vi "FocalSpot.vi"(7 "Racine chemin de sauvegarde":path=path "C:/Users/loa/Documents/DONNEES MANIP GAZ/Hiver 2015") -> ()   [LabVIEW 2014]
uses:
  <vilib>/addons/PixeLINK/Low Level Functions/ACQUISITION.llb/TDPU-Acquisition-StreamState.ctl
  <vilib>/addons/PixeLINK/Low Level Functions/CAMERA_FEATURES.llb/TDPU-CameraFeatures-FeatureIds.ctl
  <vilib>/addons/PixeLINK/Low Level Functions/CAMERA_FEATURES.llb/TDPU-CameraFeatures-FeatureFlags.ctl
  <vilib>/Platform/TimedLoop/XDataNode/timing_clust.ctl
  <vilib>/Platform/TimedLoop/XDataNode/nitl_modes.ctl
  <vilib>/Platform/TimedLoop/XDataNode/wakeup.ctl
  <vilib>/platform/TimedLoop/XDataNode/XDataNode.xnode
  <vilib>/Platform/TimedLoop/XDataNode/XDNodeRunTimeDep.lvlib
panel:
  in  "Transmission":dbl=0.5
  out "Intensity (measured)\nx10^18 W/cm²":dbl=2.0
  out "Div":dbl
  in  "Automatic\nfolder naming":bool=TRUE
  in  "Imager":u32(ring) items=["Cam 0"=953000197]
  out "?":dbl[][](graph)
  out "?":dbl[][](graph)
  in  "Background \nsubstraction":bool
  out "Intensity (gaussian)\nx10^18 W/cm²":dbl=2.0
  out "Peak power (TW)":dbl=2.0
  out "FWHM y (µm)":dbl=2.0
  out "FWHM x (µm)":dbl=2.0
  in  "Duration FWHM (fs)":dbl=4.5
  in  "Pulse Energy (mJ)":dbl=5.0
  in  "Calibration µm/px":dbl=0.5
  out "Error OUT 2":errorcluster
  out "Error OUT":errorcluster
  out "Saturating?":bool
  out "Average":dbl
  out "Std Dev":dbl
  in  "Overwrite?":bool
  in  "Snap current Data":bool
  in  "Save Data":bool
  out "Warning":bool
  out "Message":string
  in  "Indice":u32
  in  "Nom du fichier":string="tir"
  in  "Mode de Sauvegarde":u16(ring)=1 items=["Manuel", "Automatique"]
  out "Max Val":u16
  out "Captured Image":dbl[][](graph)
  out "Waiting for Trigger":bool
  in  "Continuous Grab":bool
  in  "Snap Next frame":bool
  out "Camera Handle":u32
  in  "Stop Grab\n(Insistez!)":bool
  in  "Trigger Type":enum16{"Free Running", "Software", "Hardware"}(ring)
  in  "Trigger Polarity":enum16{"Positive", "Negative"}(ring)
  in  "Refresh Trigger":bool
  in  "Exposure Time":dbl(slide) min=6.350000330712646e-05 max=10.0 scale=6.350000330712646e-05..10.0
  in  "stop":bool
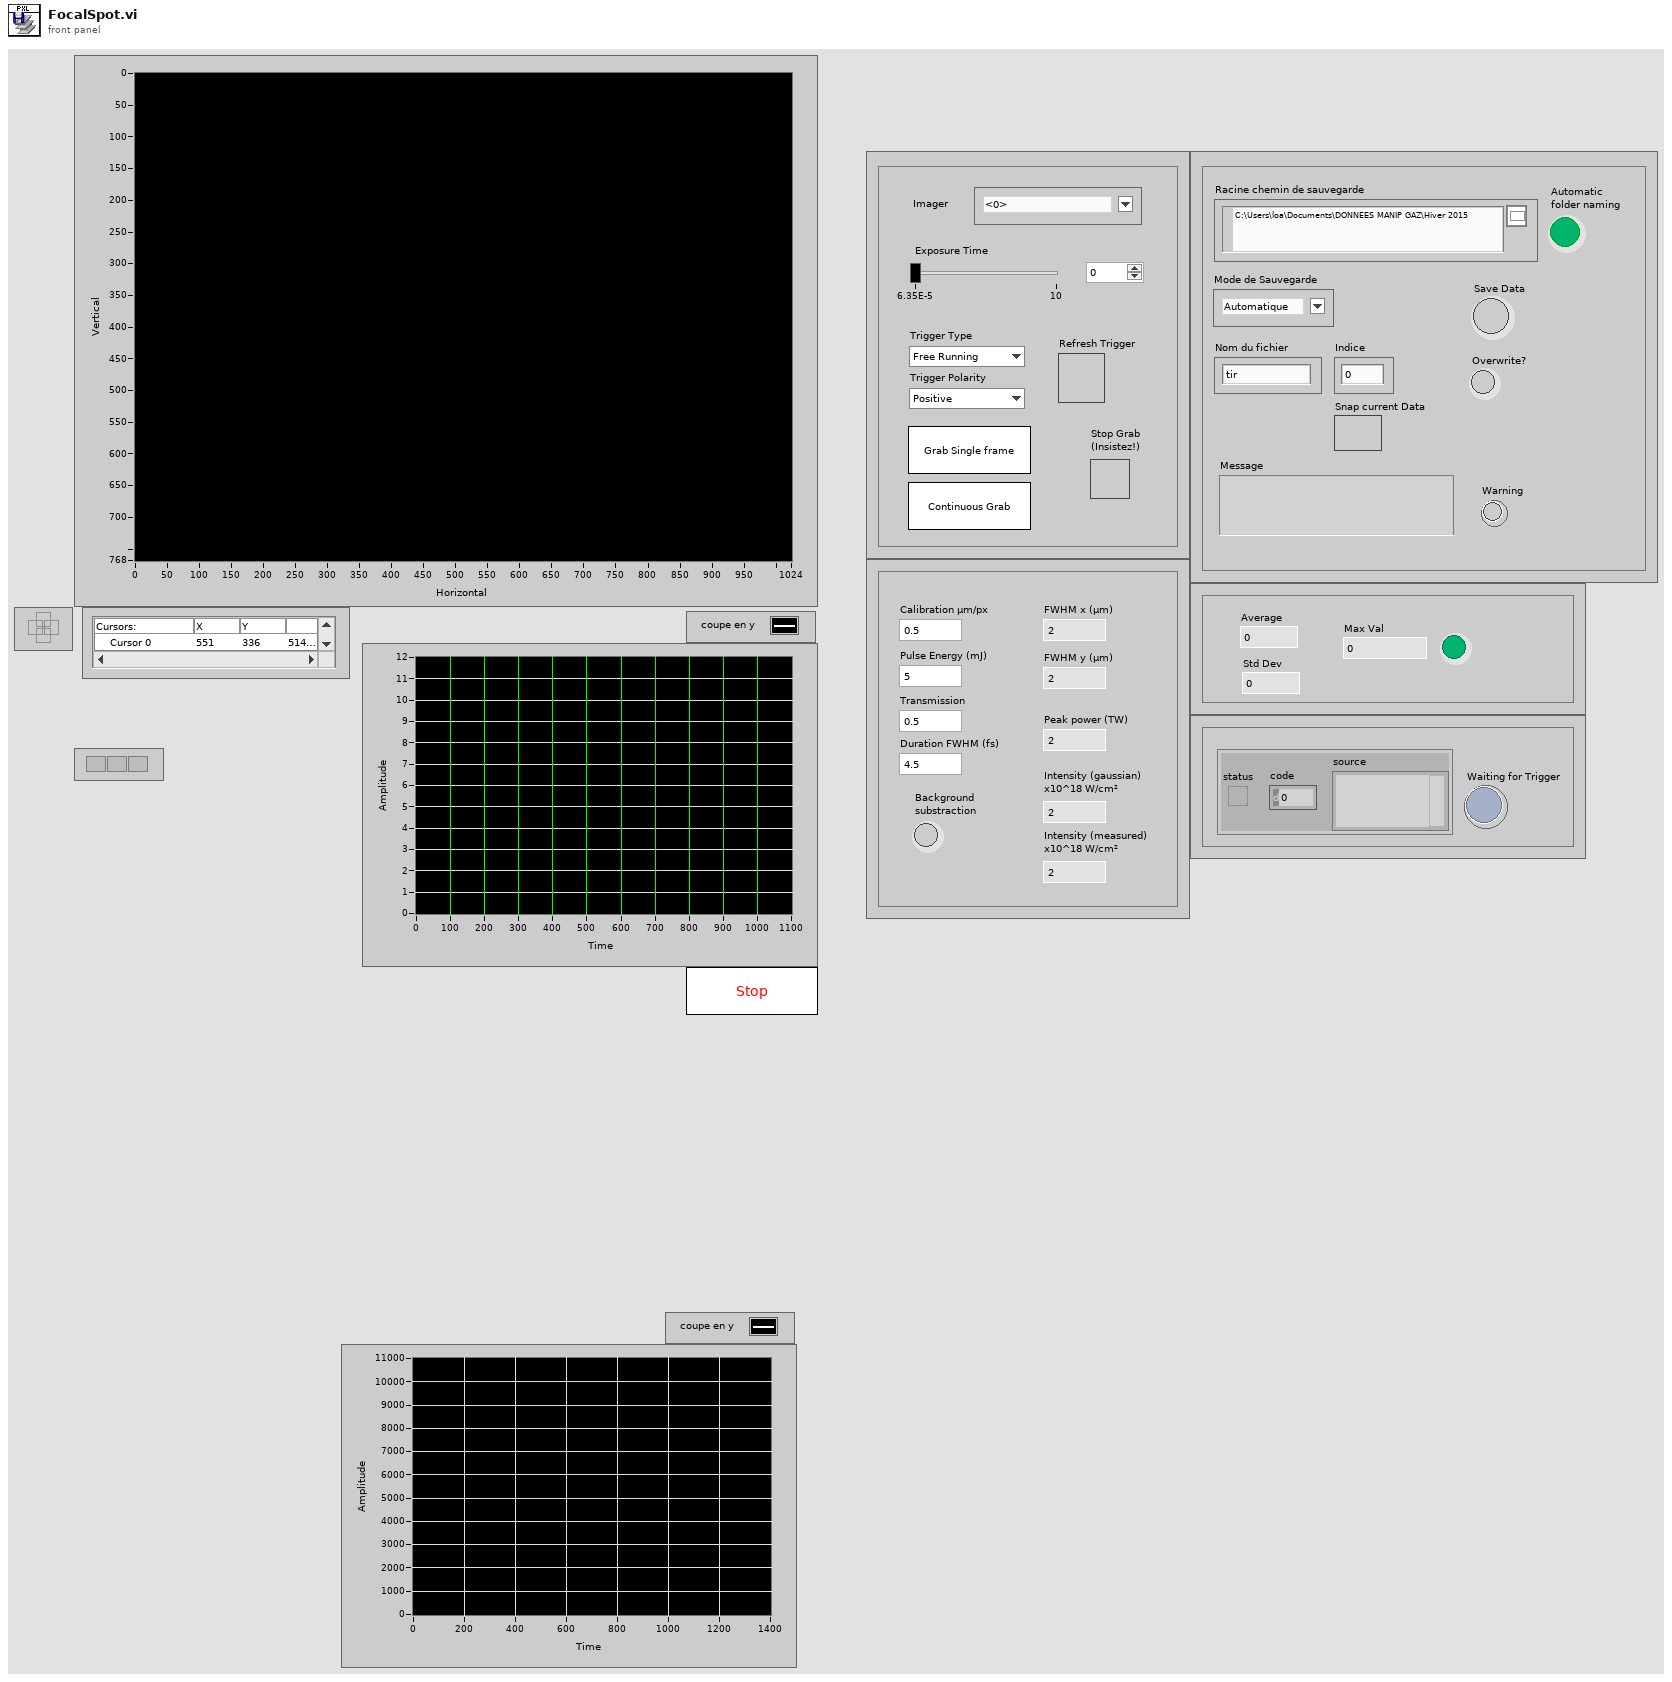
[diagram p1: front panel]
types:
  T1 = typedef "TDPU-Acquisition-StreamState.ctl" = u32
  T2 = typedef "TDPU-CameraFeatures-FeatureFlags.ctl" = u32
  T3 = typedef "TDPU-CameraFeatures-FeatureIds.ctl" = u32
  T4 = typedef "XDNodeRunTimeDep.lvlib/timing_clust.ctl" = cluster{"Expected End [f-1]":u64, "Actual End [f-1]":u64, "Finished Late? [f-1]":bool, "Expected End [i-1]":u64, "Actual End [i-1]":u64, "Finished Late? [i-1]":bool, "Expected Start [i]":u64, "Actual Start [i]":u64, "Expected Start [f]":u64, "Actual Start [f]":u64, "Source Name":string, "Structure Name":string, "Period":i64, "Deadline":i64, "Offset":i64, "Start":i64, "Priority":i32, "Timeout":i32, "Mode":T5, "Wakeup Reason":T6, "Error":errorcluster, "Source Type":string, "Secondary Source Type":string, "Global End Time":u64, "Global Start Time":u64, "Frame Duration":u64, "Iteration Duration":u64, "Assigned CPU":i32, "I/O Scan Engine Mode":u32}
  T5 = typedef "XDNodeRunTimeDep.lvlib/nitl_modes.ctl" = enum32{"No Change", "Process missed periods, maintain original phase", "Discard missed periods, maintain original phase", "Process missed periods, ignore original phase", "Discard missed periods, ignore original phase"}
  T6 = typedef "XDNodeRunTimeDep.lvlib/wakeup.ctl" = enum32{"Normal", "Aborted", "Asynchronous wakeup", "Timing source error", "Timed loop error", "Timeout"}
  T7 = typedef "LVStringsAndValuesArrayTypeDef_U32.ctl" = cluster{"String":string, "Value":u32}[]
  T8 = typedef "TDPU-Identification-Camera_Info.ctl" = cluster{"VendorName":string, "ModelName":string, "Description":string, "SerialNumber":string, "FirmwareVersion":string, "FPGAVersion":string, "CameraName":string}
  T9 = typedef "TDPU-Acquisition-Frame_Desc.ctl" = cluster{"uSize":u32, "fFrameTime":dbl, "uFrameNumber":u32, "Brightness":cluster{"fValue":dbl}, "AutoExposure":cluster{"fValue":dbl}, "Sharpness":cluster{"fValue":dbl}, "WhiteBalance":cluster{"fValue":dbl}, "Hue":cluster{"fValue":dbl}, "Saturation":cluster{"fValue":dbl}, "Gamma":cluster{"fValue":dbl}, "Shutter":cluster{"fValue":dbl}, "Gain":cluster{"fValue":dbl}, "Iris":cluster{"fValue":dbl}, "Focus":cluster{"fValue":dbl}, "Temperature":cluster{"fValue":dbl}, "Trigger":cluster{"fMode":dbl, "fType":dbl, "fPolarity":dbl, "fDelay":dbl, "fParameter":dbl}, "Zoom":cluster{"fValue":dbl}, "Pan":cluster{"fValue":dbl}, "Tilt":cluster{"fValue":dbl}, "OpticalFilter":cluster{"fValue":dbl}, "GPIO":cluster{"fMode":dbl[], "fPolarity":dbl[], "fParameter1":dbl[], "fParameter2":dbl[], "fParameter3":dbl[]}, "FrameRate":cluster{"fValue":dbl}, "ROI":cluster{"fLeft":dbl, "fTop":dbl, "fWidth":dbl, "fHeight":dbl}, "Flip":cluster{"fHorizontal":dbl, "fVertical":dbl}, "PixelAddressingValue":cluster{"fValue":dbl}, "PixelFormat":cluster{"fValue":dbl}, "ExtendedShutter":cluster{"fKneePoint":dbl[]}, "AutoROI":cluster{"fLeft":dbl, "fTop":dbl, "fWidth":dbl, "fHeight":dbl}, "WhiteShading":cluster{"fRedGain":dbl, "fGreenGain":dbl, "fBlueGain":dbl}, "Rotate":cluster{"fValue":dbl}, "PixelAddressingMode":cluster{"fValue":dbl}}
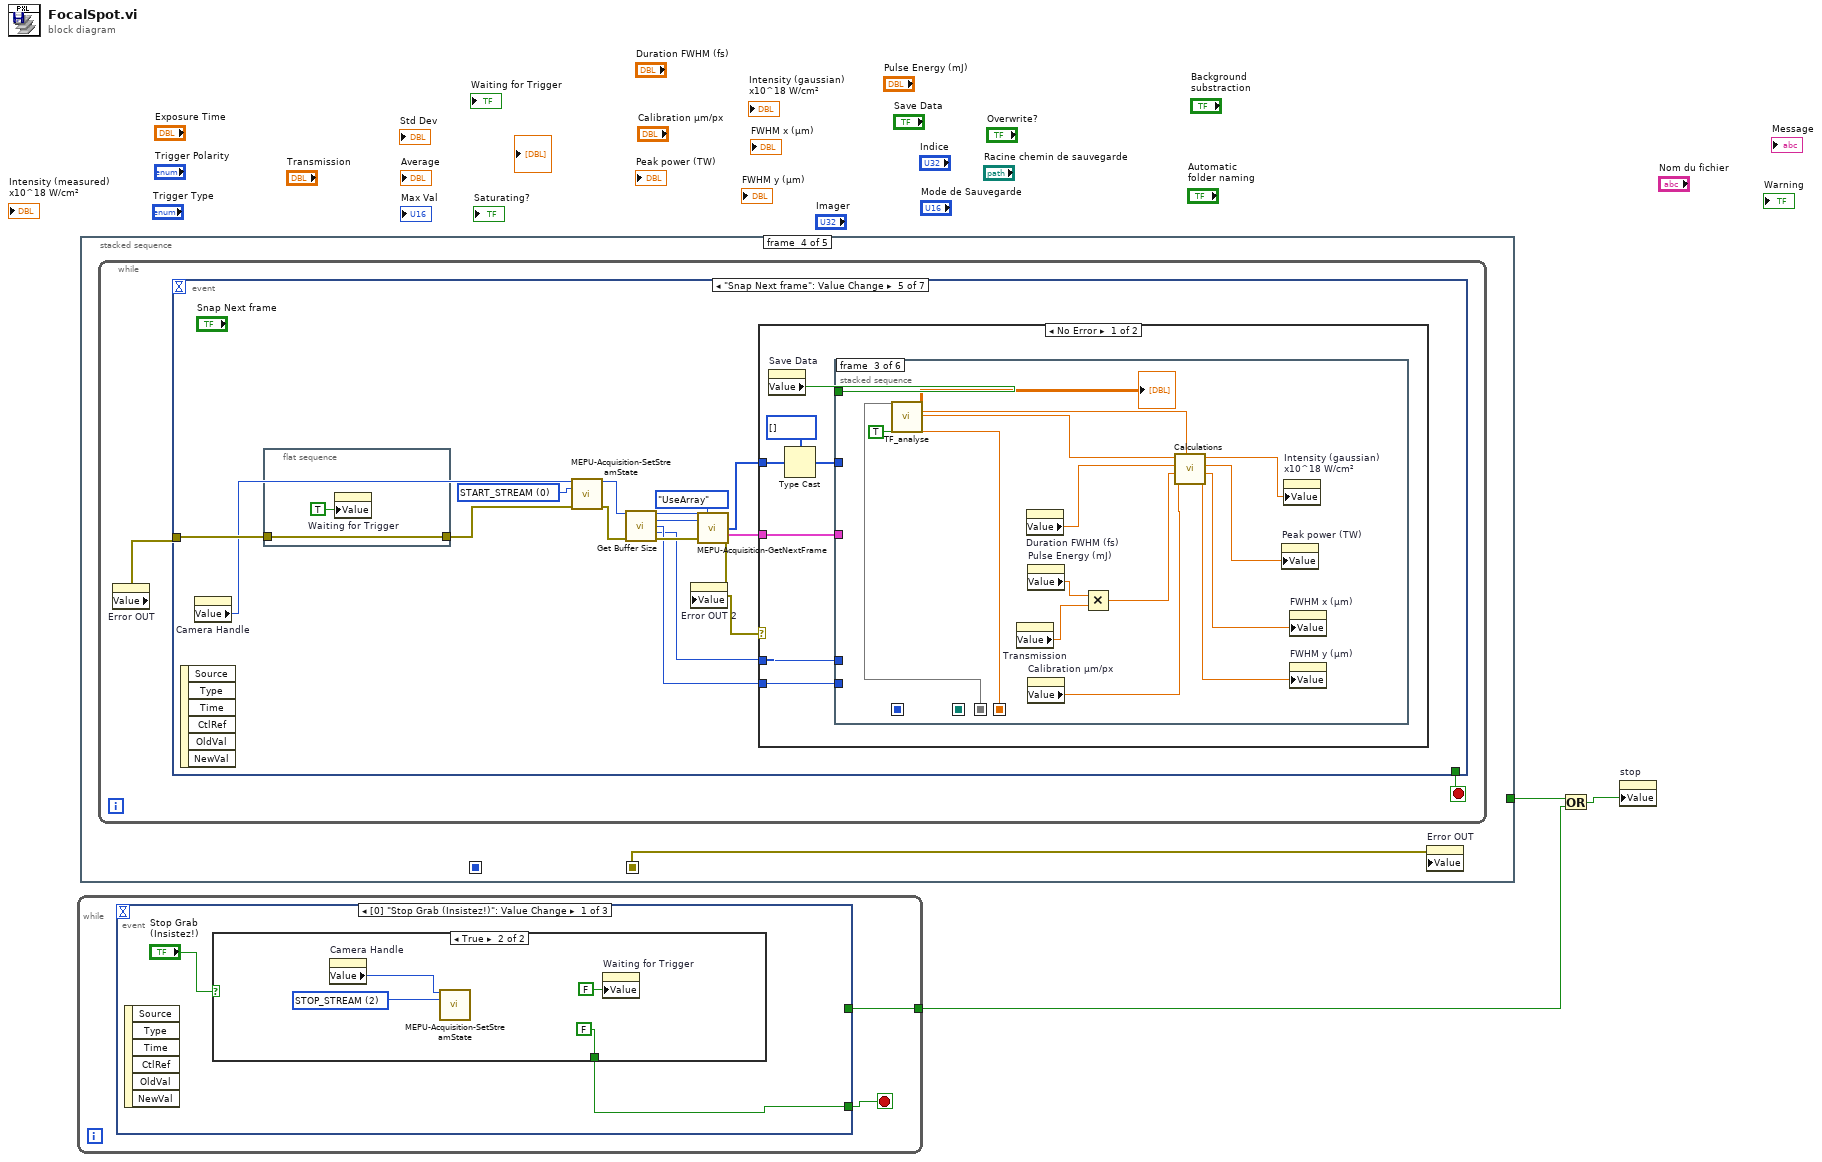
[diagram p0: block diagram]
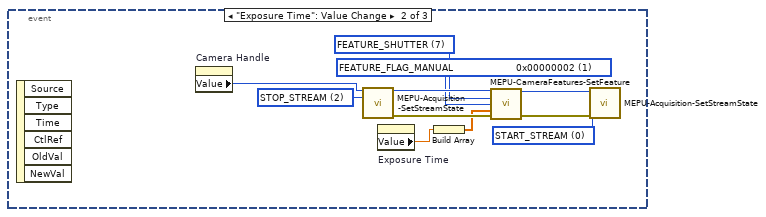
[diagram p3: hidden frame]
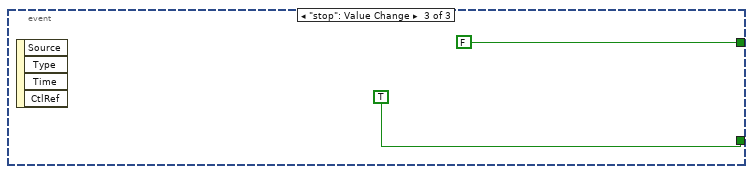
[diagram p4: hidden frame]
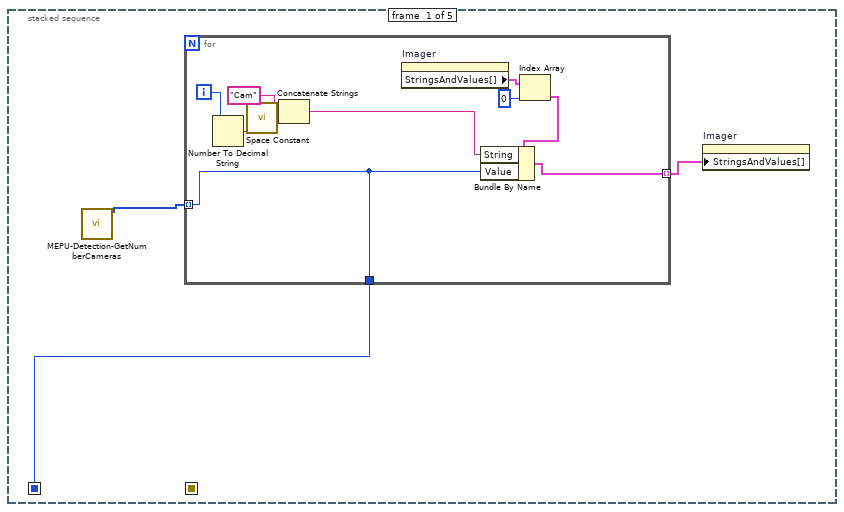
[diagram p5: hidden frame]
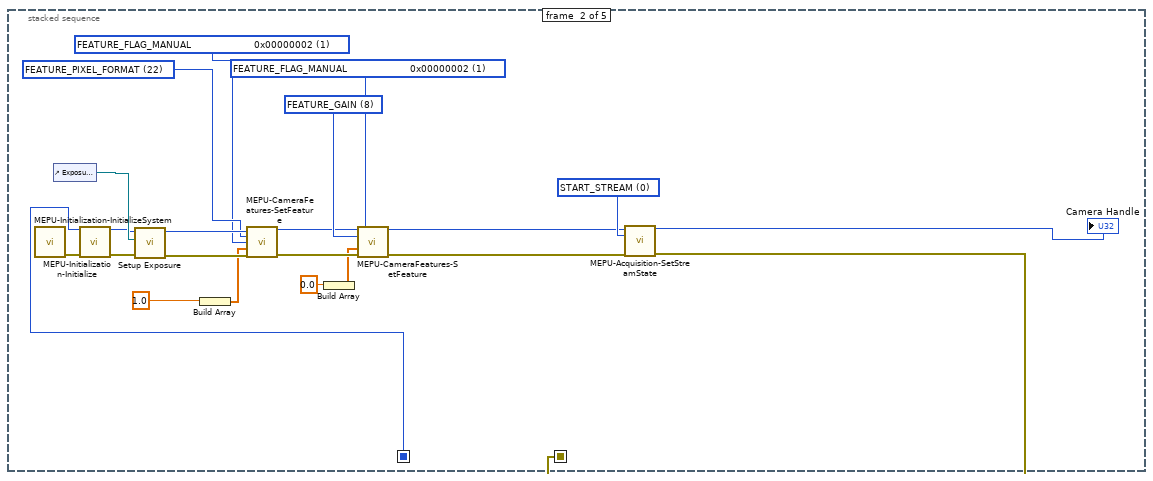
[diagram p6: hidden frame]
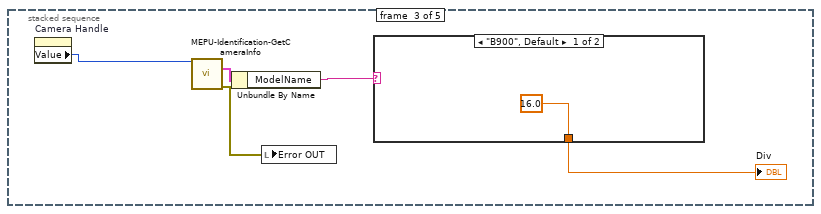
[diagram p7: hidden frame]
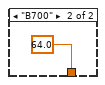
[diagram p8: hidden frame]
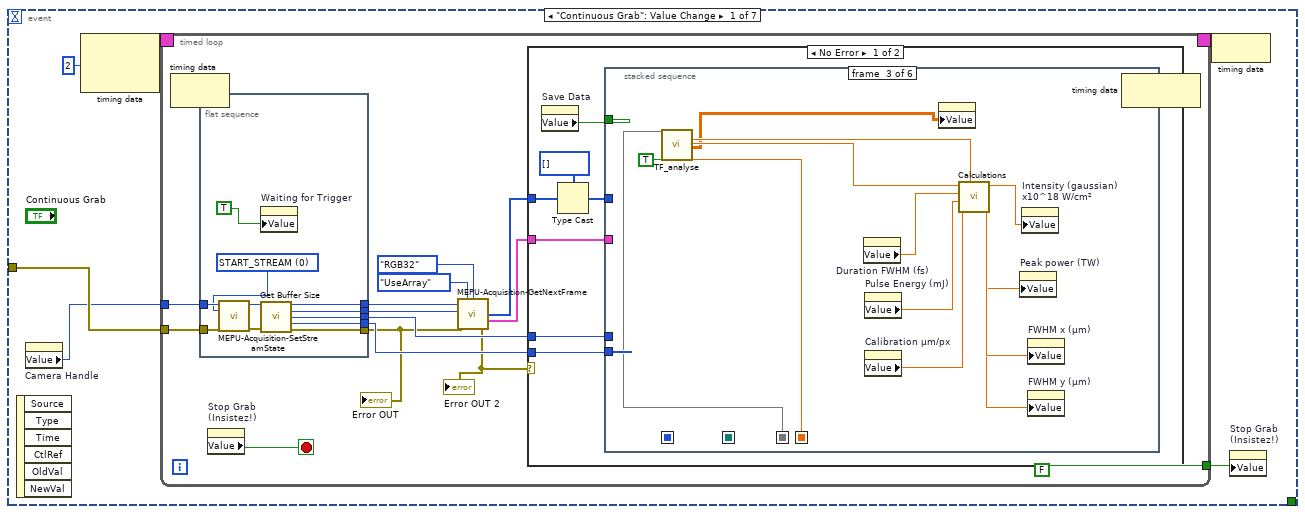
[diagram p9: hidden frame]
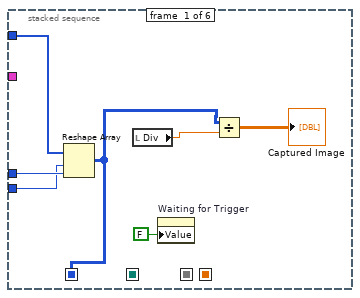
[diagram p10: hidden frame]
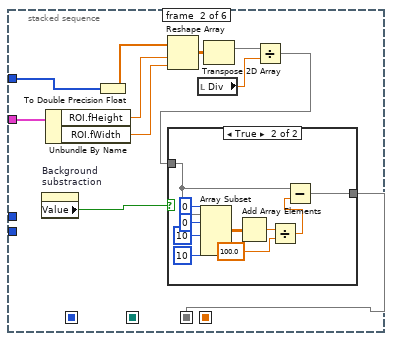
[diagram p11: hidden frame]
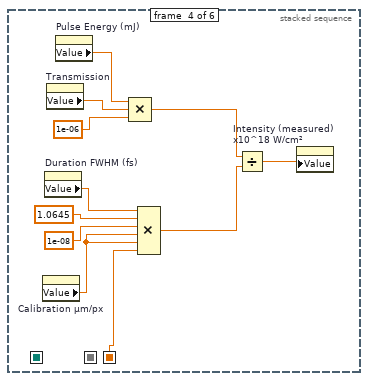
[diagram p13: hidden frame]
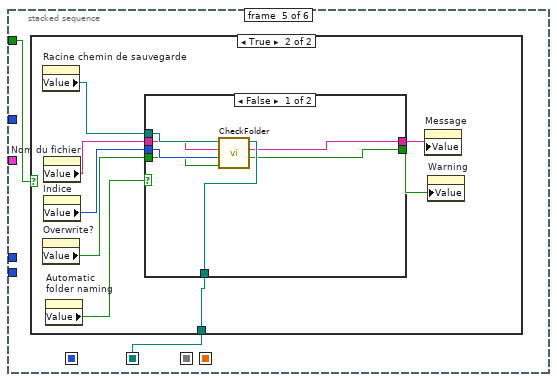
[diagram p14: hidden frame]
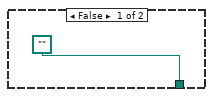
[diagram p15: hidden frame]
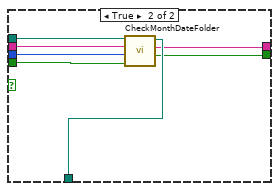
[diagram p16: hidden frame]
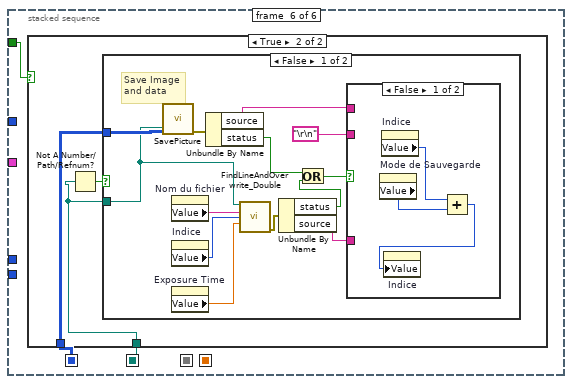
[diagram p17: hidden frame]
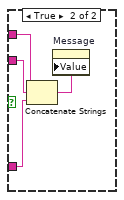
[diagram p19: hidden frame]
diagram:
  n1 = while {
    tunnel: [w4] -> w2
    stop <- w5 stop-if-true
    n2 = event shown="[0] \"Stop Grab (Insistez!)\": Value Change" {
      selector: _ -> [_ _ _]
      dyn-events: _ -> [_ _ _]
      timeout: _ -> [_ _ _]
      tunnel: [w6 _ TRUE] -> w5
      tunnel: [_ _ FALSE] -> w4
      event "Stop Grab\n(Insistez!)": Value Change {
        n3 = event-data() -> ()  [unwired: 1 in, 6 out]
        n4 = case shown="True" "Stop Grab\n(Insistez!)" {
          tunnel: [_ FALSE] -> w6
          frame False {
          }
          frame True {
            w11 = T1 2 items=["START_STREAM", "PAUSE_STREAM", "STOP_STREAM"] ("uStreamState IN")
            n5 = property on="Camera Handle" class="DigNum (strict)"() -> ("Value"=w9:u32)  [unwired: 2 in, 2 out]
            n6 = call <vilib>:"MEPU-Acquisition-SetStreamState.vi"("hCamera IN"=w9, "uStreamState IN"=w11) -> ()  [unwired: 12 in, 2 out]
            n7 = property on="Waiting for Trigger" class="Bool (strict)"("Value"=FALSE ("Waiting for Trigger")) -> ()  [unwired: 2 in, 2 out]
          }
        }
      }
      event "Exposure Time": Value Change {
        w22 = T1 0 items=["START_STREAM", "PAUSE_STREAM", "STOP_STREAM"] ("uStreamState IN")
        w21 = T1 2 items=["START_STREAM", "PAUSE_STREAM", "STOP_STREAM"] ("uStreamState IN")
        w14 = T2 1 items=["FEATURE_FLAG_PRESENCE                 0x00000001", "FEATURE_FLAG_MANUAL                     0x00000002", "FEATURE_FLAG_AUTO                         0x00000004", "FEATURE_FLAG_ONEPUSH                   0x00000008", "FEATURE_FLAG_OFF                            0x00000010", "FEATURE_FLAG_DESC_SUPPORTED    0x00000020", "FEATURE_FLAG_READ_ONLY               0x00000040"] ("uFlags IN")
        w13 = T3 7 items=["FEATURE_BRIGHTNESS", "FEATURE_EXPOSURE", "FEATURE_SHARPNESS", "FEATURE_WHITE_BAL", "FEATURE_HUE", "FEATURE_SATURATION", "FEATURE_GAMMA", "FEATURE_SHUTTER", "FEATURE_GAIN", "FEATURE_IRIS", "FEATURE_FOCUS", "FEATURE_TEMPERATURE", "FEATURE_TRIGGER", "FEATURE_ZOOM", "FEATURE_PAN", "FEATURE_TILT", "FEATURE_OPT_FILTER", "FEATURE_GPIO", "FEATURE_FRAME_RATE", "FEATURE_ROI", "FEATURE_FLIP", "FEATURE_PIXEL_ADDRESSING", "FEATURE_PIXEL_FORMAT", "FEATURE_EXTENDED_SHUTTER", "FEATURE_AUTO_ROI", "FEATURE_LOOKUP_TABLE", "FEATURE_MEMORY_CHANNEL", "FEATURE_WHITE_SHADING", "FEATURE_ROTATE", "FEATURE_IMAGER_CLK_DIVISOR", "FEATURE_TRIG_WITH_CNTRLD_LIGHT", "FEATURE_MAX_PIXEL_SIZE"] ("uFeatureId IN")
        n8 = event-data() -> ()  [unwired: 1 in, 6 out]
        n9 = property on="Camera Handle" class="DigNum (strict)"() -> ("Value"=w12:u32)  [unwired: 2 in, 2 out]
        n10 = call <vilib>:"MEPU-Acquisition-SetStreamState.vi"("hCamera IN"=w12, "uStreamState IN"=w21) -> ("hCamera OUT"=w17:u32, "Error OUT"=w20:errorcluster)  [unwired: 12 in]
        n11 = property on="Exposure Time" class="Slide (strict)"() -> ("Value"=w15:dbl)  [unwired: 2 in, 2 out]
        n12 = Build Array(w15) -> (w16:dbl[])
        n13 = call <vilib>:"MEPU-CameraFeatures-SetFeature.vi"("hCamera IN"=w17, "uFeatureId IN"=w13, "uFlags IN"=w14, "pParms IN"=w16, "Error IN"=w20) -> ("hCamera OUT"=w18:u32, "Error OUT"=w19:errorcluster)  [unwired: 9 out]
        n14 = call <vilib>:"MEPU-Acquisition-SetStreamState.vi"("hCamera IN"=w18, "uStreamState IN"=w22, "Error IN"=w19) -> ()  [unwired: 11 in, 2 out]
      }
      event "stop": Value Change {
        n15 = event-data() -> ()  [unwired: 1 in, 4 out]
      }
    }
  }
  n16 = stacked-sequence {
    seq-local: [_ w48 _ _ _] -> [_ _ _ w67 _]
    seq-local: [w25 _ _ _ _] -> [_ w38 _ _ _]
    tunnel: [_ _ _ _ TRUE] -> w3
    frame #0 {
      n17 = call <vilib>:"MEPU-Detection-GetNumberCameras.vi"() -> ("LV_SerialNumbers OUT"=w27:u32[])  [unwired: 13 in, 2 out]
      n18 = for {
        tunnel: w27 -> [w28] mode=indexing
        tunnel: [w33] -> w26 mode=indexing
        tunnel: [w28] -> w25
        i -> [w31]
        n19 = Number To Decimal String(number=w31) -> (decimal integer string=w29:string)  [unwired: 1 in]
        n20 = call <vilib>:"Space Constant.vi"() -> ("String"=w30:string)
        n21 = Concatenate Strings("Cam", w30, w29) -> (w34:string)
        n22 = property on="Imager" class="Ring (strict)"() -> ("StringsAndValues[]"=w37:T7)  [unwired: 2 in, 2 out]
        n23 = Index Array(array=w37, index=0) -> (element=w35:cluster{"String":string, "Value":u32})
        n24 = Bundle By Name(cluster=w35, "String"=w34, "Value"=w28) -> (w33:cluster{"String":string, "Value":u32})
      }
      n25 = property on="Imager" class="Ring (strict)"("StringsAndValues[]"=w26) -> ()  [unwired: 2 in, 2 out]
    }
    frame #1 {
      w43 = T2 1 items=["FEATURE_FLAG_PRESENCE                 0x00000001", "FEATURE_FLAG_MANUAL                     0x00000002", "FEATURE_FLAG_AUTO                         0x00000004", "FEATURE_FLAG_ONEPUSH                   0x00000008", "FEATURE_FLAG_OFF                            0x00000010", "FEATURE_FLAG_DESC_SUPPORTED    0x00000020", "FEATURE_FLAG_READ_ONLY               0x00000040"] ("uFlags IN")
      w42 = T3 8 items=["FEATURE_BRIGHTNESS", "FEATURE_EXPOSURE", "FEATURE_SHARPNESS", "FEATURE_WHITE_BAL", "FEATURE_HUE", "FEATURE_SATURATION", "FEATURE_GAMMA", "FEATURE_SHUTTER", "FEATURE_GAIN", "FEATURE_IRIS", "FEATURE_FOCUS", "FEATURE_TEMPERATURE", "FEATURE_TRIGGER", "FEATURE_ZOOM", "FEATURE_PAN", "FEATURE_TILT", "FEATURE_OPT_FILTER", "FEATURE_GPIO", "FEATURE_FRAME_RATE", "FEATURE_ROI", "FEATURE_FLIP", "FEATURE_PIXEL_ADDRESSING", "FEATURE_PIXEL_FORMAT", "FEATURE_EXTENDED_SHUTTER", "FEATURE_AUTO_ROI", "FEATURE_LOOKUP_TABLE", "FEATURE_MEMORY_CHANNEL", "FEATURE_WHITE_SHADING", "FEATURE_ROTATE", "FEATURE_IMAGER_CLK_DIVISOR", "FEATURE_TRIG_WITH_CNTRLD_LIGHT", "FEATURE_MAX_PIXEL_SIZE"] ("uFeatureId IN")
      w51 = T2 1 items=["FEATURE_FLAG_PRESENCE                 0x00000001", "FEATURE_FLAG_MANUAL                     0x00000002", "FEATURE_FLAG_AUTO                         0x00000004", "FEATURE_FLAG_ONEPUSH                   0x00000008", "FEATURE_FLAG_OFF                            0x00000010", "FEATURE_FLAG_DESC_SUPPORTED    0x00000020", "FEATURE_FLAG_READ_ONLY               0x00000040"] ("uFlags IN")
      w52 = T3 22 items=["FEATURE_BRIGHTNESS", "FEATURE_EXPOSURE", "FEATURE_SHARPNESS", "FEATURE_WHITE_BAL", "FEATURE_HUE", "FEATURE_SATURATION", "FEATURE_GAMMA", "FEATURE_SHUTTER", "FEATURE_GAIN", "FEATURE_IRIS", "FEATURE_FOCUS", "FEATURE_TEMPERATURE", "FEATURE_TRIGGER", "FEATURE_ZOOM", "FEATURE_PAN", "FEATURE_TILT", "FEATURE_OPT_FILTER", "FEATURE_GPIO", "FEATURE_FRAME_RATE", "FEATURE_ROI", "FEATURE_FLIP", "FEATURE_PIXEL_ADDRESSING", "FEATURE_PIXEL_FORMAT", "FEATURE_EXTENDED_SHUTTER", "FEATURE_AUTO_ROI", "FEATURE_LOOKUP_TABLE", "FEATURE_MEMORY_CHANNEL", "FEATURE_WHITE_SHADING", "FEATURE_ROTATE", "FEATURE_IMAGER_CLK_DIVISOR", "FEATURE_TRIG_WITH_CNTRLD_LIGHT", "FEATURE_MAX_PIXEL_SIZE"] ("uFeatureId IN")
      w58 = T1 0 items=["START_STREAM", "PAUSE_STREAM", "STOP_STREAM"] ("uStreamState IN")
      n26 = call <vilib>:"MEPU-Initialization-InitializeSystem.vi"() -> ("Error OUT"=w59:errorcluster)  [unwired: 15 in]
      n27 = control-ref of="Exposure Time"() -> (w57:refnum<vi>)
      n28 = call <vilib>:"MEPU-Initialization-Initialize.vi"("uSerialNumber IN"=w38, "Error IN"=w59) -> ("phCamera OUT"=w56:u32, "Error OUT"=w55:errorcluster)  [unwired: 11 in, 1 out]
      n29 = call "Setup Exposure.vi"("Error IN"=w55, "Shutter"=w57, "hCamera IN"=w56) -> ("Error OUT"=w54:errorcluster, "phCamera OUT"=w53:u32)  [unwired: 7 in]
      n30 = Build Array(1.0) -> (w49:dbl[])
      n31 = call <vilib>:"MEPU-CameraFeatures-SetFeature.vi"("hCamera IN"=w53, "uFeatureId IN"=w52, "uFlags IN"=w51, "pParms IN"=w49, "Error IN"=w54) -> ("hCamera OUT"=w41:u32, "Error OUT"=w46:errorcluster)  [unwired: 8 in, 1 out]
      n32 = Build Array(0.0) -> (w44:dbl[])
      n33 = call <vilib>:"MEPU-CameraFeatures-SetFeature.vi"("hCamera IN"=w41, "uFeatureId IN"=w42, "uFlags IN"=w43, "pParms IN"=w44, "Error IN"=w46) -> ("hCamera OUT"=w40:u32, "Error OUT"=w39:errorcluster)  [unwired: 8 in, 1 out]
      n34 = call <vilib>:"MEPU-Acquisition-SetStreamState.vi"("hCamera IN"=w40, "uStreamState IN"=w58, "Error IN"=w39) -> ("hCamera OUT"=→"Camera Handle":u32, "Error OUT"=w48:errorcluster)  [unwired: 11 in]
    }
    frame #2 {
      n35 = property on="Camera Handle" class="DigNum (strict)"() -> ("Value"=w63:u32)  [unwired: 2 in, 2 out]
      n36 = call <vilib>:"MEPU-Identification-GetCameraInfo.vi"("hCamera IN"=w63) -> ("pLVCameraInfo OUT"=w64:T8, "Error OUT"=w60:errorcluster)  [unwired: 12 in, 1 out]
      n37 = Unbundle By Name(w64) -> ("ModelName"=w62:string)
      n38 = local write "Error OUT"(w60) -> ()
      n39 = case shown="\"B900\", Default" w62 {
        tunnel: [16.0 64.0] -> w61
        frame "B900", Default {
        }
        frame "B700" {
        }
      }
      "Div" <- w61
    }
    frame #3 {
      n40 = while {
        stop <- w69 stop-if-true
        n41 = property on="Error OUT" class="Clust (strict)"() -> ("Value"=w68:errorcluster)  [unwired: 2 in, 2 out]
        n42 = event shown="[4] \"Snap Next frame\": Value Change" {
          selector: _ -> [_ _ _ _ _ _ _]
          dyn-events: _ -> [_ _ _ _ _ _ _]
          timeout: _ -> [_ _ _ _ _ _ _]
          tunnel: w68 -> [w75 _ _ w229 w247 _ _]
          tunnel: [_ _ TRUE _ _ _ _] -> w69
          event "Continuous Grab": Value Change {
            n43 = event-data() -> ()  [unwired: 1 in, 6 out]
            n44 = property on="Camera Handle" class="DigNum (strict)"() -> ("Value"=w70:u32)  [unwired: 2 in, 2 out]
            n45 = node-c288(i64 2 ("Period")) -> (w74:T4)  [unwired: 1 in]
            n46 = timed-loop {
              timing: w74 -> [_]
              timing-out: [_] -> w73
              tunnel: w70 -> [w89]
              tunnel: w75 -> [w83]
              tunnel: [FALSE] -> w71
              stop <- w80 stop-if-true
              n47 = node-c288() -> ()  [unwired: 1 in, 1 out]
              n48 = flat-sequence {
                tunnel: w89 -> [w202]
                tunnel: [w211] -> w88
                tunnel: [w210] -> w87
                tunnel: [w209] -> w78
                tunnel: w83 -> [w205]
                tunnel: [w208] -> w82
                tunnel: [w207] -> w81
                frame #0 {
                  w201 = T1 0 items=["START_STREAM", "PAUSE_STREAM", "STOP_STREAM"] ("uStreamState IN")
                  n49 = call <vilib>:"MEPU-Acquisition-SetStreamState.vi"("hCamera IN"=w202, "uStreamState IN"=w201, "Error IN"=w205) -> ("hCamera OUT"=w203:u32, "Error OUT"=w204:errorcluster)  [unwired: 11 in]
                  n50 = property on="Waiting for Trigger" class="Bool (strict)"("Value"=TRUE ("Waiting for Trigger")) -> ()  [unwired: 2 in, 2 out]
                  n51 = call "Get Buffer Size.vi"("phCamera IN"=w203, "Error IN"=w204) -> ("phCamera OUT"=w211:u32, "uBufferSize OUT"=w210:u32, "uWidth OUT"=w208:u32, "uHeight OUT"=w207:u32, "Error OUT"=w209:errorcluster)  [unwired: 8 in, 1 out]
                }
              }
              n52 = property on="Stop Grab\n(Insistez!)" class="Bool (strict)"() -> ("Value"=w80:bool)  [unwired: 2 in, 2 out]
              n53 = call <vilib>:"MEPU-Acquisition-GetNextFrame.vi"("hCamera IN"=w88, "Mode IN"=enum16{"UseArray", "UsePointer"}."UseArray", "OutputMode IN"=enum16{"Default", "RGB24", "RGB32"}."RGB32", "uBufferSize IN"=w87, "Error IN"=w78) -> ("Data OUT"=w84:u8[], "pDescriptor"=w76:T9, "Error OUT"=w77:errorcluster)  [unwired: 6 in, 2 out]
              "Error OUT 2" <- w77
              n54 = case shown="No Error" w77 {
                tunnel: w84 -> [w96 _]
                tunnel: w82 -> [w93 _]
                tunnel: w81 -> [w92 _]
                tunnel: w76 -> [w90 _]
                frame No Error {
                  n55 = property on="Save Data" class="Bool (strict)"() -> ("Value"=w91:bool)  [unwired: 2 in, 2 out]
                  n56 = Type Cast(type=u16[] [] ("Data OUT"), x=w96) -> (*(type *) &x=w94:u16[])
                  n57 = stacked-sequence {
                    seq-local: [_ _ _ _ w151 _] -> [_ _ _ _ _ w177]
                    seq-local: [_ w108 _ _ _ _] -> [_ _ w137 _ _ _]
                    seq-local: [w99 _ _ _ _ _] -> [_ _ _ _ _ w175]
                    seq-local: [_ _ w126 _ _ _] -> [_ _ _ w139 _ _]
                    tunnel: w94 -> [w103 w111 _ _ _ _]
                    tunnel: w93 -> [w102 _ _ _ _ _]
                    tunnel: w92 -> [w101 _ _ _ _ _]
                    tunnel: w91 -> [_ _ _ _ w150 w176]
                    tunnel: w90 -> [_ w114 _ _ _ _]
                    frame #0 {
                      n58 = Reshape Array(w103, w101, w102) -> (w99:u16[][])
                      n59 = local read "Div"() -> (w98:dbl)
                      n60 = property on="Waiting for Trigger" class="Bool (strict)"("Value"=FALSE ("Waiting for Trigger")) -> ()  [unwired: 2 in, 2 out]
                      n61 = Divide(x=w99, y=w98) -> (x/y=→"Captured Image":dbl[][])
                    }
                    frame #1 {
                      n62 = property on="Background \nsubstraction" class="Bool (strict)"() -> ("Value"=w107:bool)  [unwired: 2 in, 2 out]
                      n63 = Unbundle By Name(w114) -> ("ROI.fHeight"=w113:dbl, "ROI.fWidth"=w112:dbl)
                      n64 = To Double Precision Float(number=w111) -> (double precision float=w109:dbl[])
                      n65 = Reshape Array(w109, w113, w112) -> (w110:dbl[][])
                      n66 = local read "Div"() -> (w105:dbl)
                      n67 = Transpose 2D Array(2D array=w110) -> (transposed array=w106:dbl[][])
                      n68 = Divide(x=w106, y=w105) -> (x/y=w104:dbl[][])
                      n69 = case shown="True" w107 {
                        tunnel: w104 -> [w115 w117]
                        tunnel: [w115 w116] -> w108
                        frame False {
                        }
                        frame True {
                          n70 = Array Subset(array=w117, index (row)=0 ("index"), length (row)=10 ("length"), index (col)=0 ("index"), length (col)=10 ("length")) -> (w121:dbl[][])
                          n71 = Add Array Elements(numeric array=w121) -> (sum=w120:dbl)
                          n72 = Divide(x=w120, y=100.0 ("sum")) -> (x/y=w118:dbl)
                          n73 = Subtract(x=w117, y=w118) -> (x-y=w116:dbl[][])
                        }
                      }
                    }
                    frame #2 {
                      n74 = call "TF_analyse.vi"("image 2D"=w137, "FLUENCE calculation"=TRUE) -> ("FWHM en x"=w132:dbl, "FWHM en y"=w133:dbl, "coupes x & y"=w127:dbl[][], "intégration totale"=w126:dbl)  [unwired: 19 in, 3 out]
                      n75 = property on="Duration FWHM (fs)" class="DigNum (strict)"() -> ("Value"=w134:dbl)  [unwired: 2 in, 2 out]
                      n76 = property on="Pulse Energy (mJ)" class="DigNum (strict)"() -> ("Value"=w135:dbl)  [unwired: 2 in, 2 out]
                      n77 = property on="Calibration µm/px" class="DigNum (strict)"() -> ("Value"=w136:dbl)  [unwired: 2 in, 2 out]
                      n78 = property class="WFGraph (strict)"("Value"=w127) -> ()  [unwired: 2 in, 2 out]
                      n79 = call "Calculations.vi"("FWHM x (px)"=w132, "Calibration µm/px"=w136, "Energy in 1 Pulse (mJ)"=w135, "Pulse Duration (fs)"=w134, "FWHM y (px)"=w133) -> ("FWHM y (µm)"=w130:dbl, "FWHM x (µm)"=w131:dbl, "Peak Power (TW)"=w129:dbl, "Integral of Perfect Gaussian (x10^18 W/cm²)"=w128:dbl)  [unwired: 3 in]
                      n80 = property on="Peak power (TW)" class="DigNum (strict)"("Value"=w129) -> ()  [unwired: 2 in, 2 out]
                      n81 = property on="Intensity (gaussian)\nx10^18 W/cm²" class="DigNum (strict)"("Value"=w128) -> ()  [unwired: 2 in, 2 out]
                      n82 = property on="FWHM x (µm)" class="DigNum (strict)"("Value"=w131) -> ()  [unwired: 2 in, 2 out]
                      n83 = property on="FWHM y (µm)" class="DigNum (strict)"("Value"=w130) -> ()  [unwired: 2 in, 2 out]
                    }
                    frame #3 {
                      n84 = property on="Calibration µm/px" class="DigNum (strict)"() -> ("Value"=w143:dbl)  [unwired: 2 in, 2 out]
                      n85 = property on="Duration FWHM (fs)" class="DigNum (strict)"() -> ("Value"=w146:dbl)  [unwired: 2 in, 2 out]
                      n86 = property on="Transmission" class="DigNum (strict)"() -> ("Value"=w148:dbl)  [unwired: 2 in, 2 out]
                      n87 = property on="Pulse Energy (mJ)" class="DigNum (strict)"() -> ("Value"=w149:dbl)  [unwired: 2 in, 2 out]
                      n88 = Compound Arithmetic op=MULTIPLY(w149, w148, 1e-06 ("Transmission")) -> (w142:dbl)
                      n89 = Compound Arithmetic op=MULTIPLY(w146, 1.0645 ("Transmission"), 1e-08 ("Transmission"), w143, w143, w139) -> (w141:dbl)
                      n90 = Divide(x=w142, y=w141) -> (x/y=w140:dbl)
                      n91 = property on="Intensity (measured)\nx10^18 W/cm²" class="DigNum (strict)"("Value"=w140) -> ()  [unwired: 2 in, 2 out]
                    }
                    frame #4 {
                      n92 = case shown="True" w150 {
                        tunnel: [path "" ("File Path") w156] -> w151
                        frame False {
                        }
                        frame True {
                          n93 = property on="Racine chemin de sauvegarde" class="Path"() -> ("Value"=w157:path)  [unwired: 2 in, 2 out]
                          n94 = property on="Overwrite?" class="Bool (strict)"() -> ("Value"=w160:bool)  [unwired: 2 in, 2 out]
                          n95 = property on="Nom du fichier" class="Str"() -> ("Value"=w158:string)  [unwired: 2 in, 2 out]
                          n96 = property on="Indice" class="DigNum (strict)"() -> ("Value"=w159:u32)  [unwired: 2 in, 2 out]
                          n97 = property on="Automatic\nfolder naming" class="Bool (strict)"() -> ("Value"=w153:bool)  [unwired: 2 in, 2 out]
                          n98 = case shown="False" w153 {
                            tunnel: w160 -> [w164 w174]
                            tunnel: w159 -> [w165 w173]
                            tunnel: w158 -> [w166 w172]
                            tunnel: w157 -> [w167 w171]
                            tunnel: [w163 w170] -> w156
                            tunnel: [w162 w169] -> w155
                            tunnel: [w161 w168] -> w154
                            frame False {
                              n99 = call "CheckFolder.vi"("Overwrite?"=w164, "Index"=w165, "File Name"=w166, "Folder Path Control"=w167) -> ("Warning"=w161:bool, "Message"=w162:string, "File Path"=w163:path)  [unwired: 5 in]
                            }
                            frame True {
                              n100 = call "CheckMonthDateFolder.vi"("Overwrite?"=w174, "Index"=w173, "File Name"=w172, "Folder Path Control"=w171) -> ("Warning"=w168:bool, "Message"=w169:string, "File Path"=w170:path)  [unwired: 5 in]
                            }
                          }
                          n101 = property on="Message" class="Str"("Value"=w155) -> ()  [unwired: 2 in, 2 out]
                          n102 = property on="Warning" class="Bool (strict)"("Value"=w154) -> ()  [unwired: 2 in, 2 out]
                        }
                      }
                    }
                    frame #5 {
                      n103 = case shown="True" w176 {
                        tunnel: w177 -> [_ w179]
                        tunnel: w175 -> [_ w178]
                        frame False {
                        }
                        frame True {
                          n104 = Not A Number/Path/Refnum?(number/path/refnum=w179) -> (NaN/Path/Refnum?=w180:bool)
                          n105 = case shown="False" w180 {
                            tunnel: w179 -> [w183 _]
                            tunnel: w178 -> [w186 _]
                            frame False {
                              # "Save Image\nand data"
                              n106 = call "SavePicture.vi"("File Path"=w183, "Image Pixels (U16)"=w186) -> ("error out"=w192:errorcluster)  [unwired: 9 in]
                              n107 = property on="Nom du fichier" class="Str"() -> ("Value"=w184:string)  [unwired: 2 in, 2 out]
                              n108 = property on="Indice" class="DigNum (strict)"() -> ("Value"=w182:u32)  [unwired: 2 in, 2 out]
                              n109 = property on="Exposure Time" class="Slide (strict)"() -> ("Value"=w181:dbl)  [unwired: 2 in, 2 out]
                              n110 = Unbundle By Name(w192) -> ("source"=w189:string, "status"=w190:bool)
                              n111 = call "FindLineAndOverwrite_Double.vi"("Exposure path"=w183, "Name"=w184, "Index"=w182, "Exposure"=w181) -> ("error out"=w185:errorcluster)  [unwired: 11 in]
                              n112 = Unbundle By Name(w185) -> ("status"=w191:bool, "source"=w193:string)
                              n113 = Or(x=w190, y=w191) -> (x .or. y?=w188:bool)
                              n114 = case shown="False" w188 {
                                tunnel: w193 -> [_ w197]
                                tunnel: w189 -> [_ w200]
                                tunnel: "\r\n" -> [_ w198]
                                frame False {
                                n115 = property on="Mode de Sauvegarde" class="Ring (strict)"() -> ("Value"=w195:u16)  [unwired: 2 in, 2 out]
                                n116 = property on="Indice" class="DigNum (strict)"() -> ("Value"=w196:u32)  [unwired: 2 in, 2 out]
                                n117 = Add(x=w196, y=w195) -> (x+y=w194:u32)
                                n118 = property on="Indice" class="DigNum (strict)"("Value"=w194) -> ()  [unwired: 2 in, 2 out]
                                }
                                frame True {
                                n119 = Concatenate Strings(w200, w198, w197) -> (w199:string)
                                n120 = property on="Message" class="Str"("Value"=w199) -> ()  [unwired: 2 in, 2 out]
                                }
                              }
                            }
                            frame True {
                            }
                          }
                        }
                      }
                    }
                  }
                }
                frame Error {
                }
              }
              n121 = node-c288() -> ()  [unwired: 1 in, 1 out]
              "Error OUT" <- w78
            }
            n122 = node-c288(w73) -> ()
            n123 = property on="Stop Grab\n(Insistez!)" class="Bool (strict)"("Value"=w71) -> ()  [unwired: 2 in, 2 out]
          }
          event "Trigger Polarity", "Trigger Type": Value Change {
            n124 = event-data() -> ()  [unwired: 1 in, 6 out]
            n125 = property on="Refresh Trigger" class="Bool"("Blinking"=TRUE) -> ()  [unwired: 2 in, 2 out]
          }
          event "stop": Value Change {
            n126 = event-data() -> ()  [unwired: 1 in, 6 out]
            n127 = property on="Refresh Trigger" class="Bool"("Blinking"=FALSE) -> ()  [unwired: 2 in, 2 out]
          }
          event "Refresh Trigger": Value Change {
            w223 = T1 2 items=["START_STREAM", "PAUSE_STREAM", "STOP_STREAM"] ("uStreamState IN")
            w224 = T1 0 items=["START_STREAM", "PAUSE_STREAM", "STOP_STREAM"] ("uStreamState IN")
            w238 = T2 1 items=["FEATURE_FLAG_PRESENCE                 0x00000001", "FEATURE_FLAG_MANUAL                     0x00000002", "FEATURE_FLAG_AUTO                         0x00000004", "FEATURE_FLAG_ONEPUSH                   0x00000008", "FEATURE_FLAG_OFF                            0x00000010", "FEATURE_FLAG_DESC_SUPPORTED    0x00000020", "FEATURE_FLAG_READ_ONLY               0x00000040"] ("uFlags IN")
            w239 = T3 12 items=["FEATURE_BRIGHTNESS", "FEATURE_EXPOSURE", "FEATURE_SHARPNESS", "FEATURE_WHITE_BAL", "FEATURE_HUE", "FEATURE_SATURATION", "FEATURE_GAMMA", "FEATURE_SHUTTER", "FEATURE_GAIN", "FEATURE_IRIS", "FEATURE_FOCUS", "FEATURE_TEMPERATURE", "FEATURE_TRIGGER", "FEATURE_ZOOM", "FEATURE_PAN", "FEATURE_TILT", "FEATURE_OPT_FILTER", "FEATURE_GPIO", "FEATURE_FRAME_RATE", "FEATURE_ROI", "FEATURE_FLIP", "FEATURE_PIXEL_ADDRESSING", "FEATURE_PIXEL_FORMAT", "FEATURE_EXTENDED_SHUTTER", "FEATURE_AUTO_ROI", "FEATURE_LOOKUP_TABLE", "FEATURE_MEMORY_CHANNEL", "FEATURE_WHITE_SHADING", "FEATURE_ROTATE", "FEATURE_IMAGER_CLK_DIVISOR", "FEATURE_TRIG_WITH_CNTRLD_LIGHT", "FEATURE_MAX_PIXEL_SIZE"] ("uFeatureId IN")
            n128 = event-data() -> ()  [unwired: 1 in, 6 out]
            n129 = property on="Camera Handle" class="DigNum (strict)"() -> ("Value"=w221:u32)  [unwired: 2 in, 2 out]
            n130 = property on="Refresh Trigger" class="Bool"("Blinking"=FALSE) -> ()  [unwired: 2 in, 2 out]
            n131 = property on="Trigger Polarity" class="Enum (strict)"() -> ("Value"=w234:enum16{"Positive", "Negative"})  [unwired: 2 in, 2 out]
            n132 = property on="Trigger Type" class="Enum (strict)"() -> ("Value"=w236:enum16{"Free Running", "Software", "Hardware"})  [unwired: 2 in, 2 out]
            n133 = To Double Precision Float(number=w234) -> (double precision float=w233:dbl)
            n134 = To Double Precision Float(number=w236) -> (double precision float=w235:dbl)
            n135 = Build Array(0.0 ("element"), w235, w233, 0.0 ("element"), 0.0 ("element")) -> (w230:dbl[])
            n136 = call <vilib>:"MEPU-Acquisition-SetStreamState.vi"("hCamera IN"=w221, "uStreamState IN"=w223, "Error IN"=w229) -> ("hCamera OUT"=w228:u32, "Error OUT"=w227:errorcluster)  [unwired: 11 in]
            n137 = call <vilib>:"MEPU-CameraFeatures-SetFeature.vi"("hCamera IN"=w228, "uFeatureId IN"=w239, "uFlags IN"=w238, "pParms IN"=w230, "Error IN"=w227) -> ("hCamera OUT"=w225:u32, "Error OUT"=w226:errorcluster)  [unwired: 9 out]
            n138 = call <vilib>:"MEPU-Acquisition-SetStreamState.vi"("hCamera IN"=w225, "uStreamState IN"=w224, "Error IN"=w226) -> ()  [unwired: 11 in, 2 out]
          }
          event "Snap Next frame": Value Change {
            w250 = T1 0 items=["START_STREAM", "PAUSE_STREAM", "STOP_STREAM"] ("uStreamState IN")
            n139 = event-data() -> ()  [unwired: 1 in, 6 out]
            n140 = property on="Camera Handle" class="DigNum (strict)"() -> ("Value"=w240:u32)  [unwired: 2 in, 2 out]
            n141 = flat-sequence {
              tunnel: w247 -> [w366]
              tunnel: [w366] -> w246
              frame #0 {
                n142 = property on="Waiting for Trigger" class="Bool (strict)"("Value"=TRUE ("Waiting for Trigger")) -> ()  [unwired: 2 in, 2 out]
              }
            }
            n143 = call <vilib>:"MEPU-Acquisition-SetStreamState.vi"("hCamera IN"=w240, "uStreamState IN"=w250, "Error IN"=w246) -> ("hCamera OUT"=w249:u32, "Error OUT"=w248:errorcluster)  [unwired: 11 in]
            n144 = call "Get Buffer Size.vi"("phCamera IN"=w249, "Error IN"=w248) -> ("phCamera OUT"=w254:u32, "uBufferSize OUT"=w252:u32, "uWidth OUT"=w243:u32, "uHeight OUT"=w242:u32, "Error OUT"=w253:errorcluster)  [unwired: 8 in, 1 out]
            n145 = call <vilib>:"MEPU-Acquisition-GetNextFrame.vi"("hCamera IN"=w254, "Mode IN"=enum16{"UseArray", "UsePointer"}."UseArray", "uBufferSize IN"=w252, "Error IN"=w253) -> ("Data OUT"=w245:u8[], "pDescriptor"=w241:T9, "Error OUT"=w244:errorcluster)  [unwired: 7 in, 2 out]
            n146 = property on="Error OUT 2" class="Clust (strict)"("Value"=w244) -> ()  [unwired: 2 in, 2 out]
            n147 = case shown="No Error" w244 {
              tunnel: w245 -> [w258 _]
              tunnel: w243 -> [w257 _]
              tunnel: w242 -> [w256 _]
              tunnel: w241 -> [w255 _]
              frame No Error {
                n148 = property on="Save Data" class="Bool (strict)"() -> ("Value"=w259:bool)  [unwired: 2 in, 2 out]
                n149 = Type Cast(type=u16[] [] ("Data OUT"), x=w258) -> (*(type *) &x=w260:u16[])
                n150 = stacked-sequence {
                  seq-local: [_ _ _ _ w316 _] -> [_ _ _ _ _ w342]
                  seq-local: [_ w273 _ _ _ _] -> [_ _ w302 _ _ _]
                  seq-local: [w264 _ _ _ _ _] -> [_ _ _ _ _ w340]
                  seq-local: [_ _ w292 _ _ _] -> [_ _ _ w307 _ _]
                  tunnel: w260 -> [w268 w277 _ _ _ _]
                  tunnel: w259 -> [_ _ _ _ w315 w341]
                  tunnel: w257 -> [w266 _ _ _ _ _]
                  tunnel: w256 -> [w265 _ _ _ _ _]
                  tunnel: w255 -> [_ w272 _ _ _ _]
                  frame #0 {
                    n151 = Reshape Array(w268, w265, w266) -> (w264:u16[][])
                    n152 = local read "Div"() -> (w263:dbl)
                    n153 = Divide(x=w264, y=w263) -> (x/y=w262:dbl[][])
                    n154 = property on="Waiting for Trigger" class="Bool (strict)"("Value"=FALSE ("Waiting for Trigger")) -> ()  [unwired: 2 in, 2 out]
                    n155 = property on="Captured Image" class="IntGraph (strict)"("Value"=w262) -> ()  [unwired: 2 in, 2 out]
                  }
                  frame #1 {
                    n156 = Unbundle By Name(w272) -> ("ROI.fHeight"=w271:dbl, "ROI.fWidth"=w270:dbl)
                    n157 = property on="Background \nsubstraction" class="Bool (strict)"() -> ("Value"=w269:bool)  [unwired: 2 in, 2 out]
                    n158 = To Double Precision Float(number=w277) -> (double precision float=w275:dbl[])
                    n159 = Reshape Array(w275, w271, w270) -> (w276:dbl[][])
                    n160 = Transpose 2D Array(2D array=w276) -> (transposed array=w274:dbl[][])
                    n161 = case shown="False" w269 {
                      tunnel: w274 -> [w278 w280]
                      tunnel: [w278 w279] -> w273
                      frame False {
                      }
                      frame True {
                        n162 = Array Subset(array=w280, index (row)=0 ("index"), length (row)=10 ("length"), index (col)=0 ("index"), length (col)=10 ("length")) -> (w284:dbl[][])
                        n163 = Add Array Elements(numeric array=w284) -> (sum=w283:dbl)
                        n164 = Divide(x=w283, y=100.0 ("sum")) -> (x/y=w281:dbl)
                        n165 = Subtract(x=w280, y=w281) -> (x-y=w279:dbl[][])
                      }
                    }
                  }
                  frame #2 {
                    n166 = call "TF_analyse.vi"("image 2D"=w302, "FLUENCE calculation"=TRUE) -> ("FWHM en x"=w298:dbl, "FWHM en y"=w299:dbl, "coupes x & y"=→"?":dbl[][], "intégration totale"=w292:dbl)  [unwired: 19 in, 3 out]
                    n167 = property on="Transmission" class="DigNum (strict)"() -> ("Value"=w289:dbl)  [unwired: 2 in, 2 out]
                    n168 = property on="Duration FWHM (fs)" class="DigNum (strict)"() -> ("Value"=w300:dbl)  [unwired: 2 in, 2 out]
                    n169 = property on="Pulse Energy (mJ)" class="DigNum (strict)"() -> ("Value"=w290:dbl)  [unwired: 2 in, 2 out]
                    n170 = property on="Calibration µm/px" class="DigNum (strict)"() -> ("Value"=w301:dbl)  [unwired: 2 in, 2 out]
                    n171 = Multiply(x=w290, y=w289) -> (x*y=w291:dbl)
                    n172 = call "Calculations.vi"("FWHM x (px)"=w298, "Calibration µm/px"=w301, "Energy in 1 Pulse (mJ)"=w291, "Pulse Duration (fs)"=w300, "FWHM y (px)"=w299) -> ("FWHM y (µm)"=w295:dbl, "FWHM x (µm)"=w296:dbl, "Peak Power (TW)"=w294:dbl, "Integral of Perfect Gaussian (x10^18 W/cm²)"=w293:dbl)  [unwired: 3 in]
                    n173 = property on="Peak power (TW)" class="DigNum (strict)"("Value"=w294) -> ()  [unwired: 2 in, 2 out]
                    n174 = property on="Intensity (gaussian)\nx10^18 W/cm²" class="DigNum (strict)"("Value"=w293) -> ()  [unwired: 2 in, 2 out]
                    n175 = property on="FWHM x (µm)" class="DigNum (strict)"("Value"=w296) -> ()  [unwired: 2 in, 2 out]
                    n176 = property on="FWHM y (µm)" class="DigNum (strict)"("Value"=w295) -> ()  [unwired: 2 in, 2 out]
                  }
                  frame #3 {
                    n177 = property on="Calibration µm/px" class="DigNum (strict)"() -> ("Value"=w308:dbl)  [unwired: 2 in, 2 out]
                    n178 = property on="Duration FWHM (fs)" class="DigNum (strict)"() -> ("Value"=w311:dbl)  [unwired: 2 in, 2 out]
                    n179 = property on="Transmission" class="DigNum (strict)"() -> ("Value"=w313:dbl)  [unwired: 2 in, 2 out]
                    n180 = property on="Pulse Energy (mJ)" class="DigNum (strict)"() -> ("Value"=w314:dbl)  [unwired: 2 in, 2 out]
                    n181 = Compound Arithmetic op=MULTIPLY(w314, w313, 1e-06 ("Transmission")) -> (w306:dbl)
                    n182 = Compound Arithmetic op=MULTIPLY(w311, 1.0645 ("Transmission"), 1e-08 ("Transmission"), w308, w308, w307) -> (w305:dbl)
                    n183 = Divide(x=w306, y=w305) -> (x/y=w304:dbl)
                    n184 = property on="Intensity (measured)\nx10^18 W/cm²" class="DigNum (strict)"("Value"=w304) -> ()  [unwired: 2 in, 2 out]
                  }
                  frame #4 {
                    n185 = case shown="True" w315 {
                      tunnel: [path "" ("File Path") w321] -> w316
                      frame False {
                      }
                      frame True {
                        n186 = property on="Racine chemin de sauvegarde" class="Path"() -> ("Value"=w322:path)  [unwired: 2 in, 2 out]
                        n187 = property on="Nom du fichier" class="Str"() -> ("Value"=w323:string)  [unwired: 2 in, 2 out]
                        n188 = property on="Indice" class="DigNum (strict)"() -> ("Value"=w324:u32)  [unwired: 2 in, 2 out]
                        n189 = property on="Overwrite?" class="Bool (strict)"() -> ("Value"=w325:bool)  [unwired: 2 in, 2 out]
                        n190 = property on="Automatic\nfolder naming" class="Bool (strict)"() -> ("Value"=w318:bool)  [unwired: 2 in, 2 out]
                        n191 = case shown="True" w318 {
                          tunnel: w325 -> [w329 w339]
                          tunnel: w324 -> [w330 w338]
                          tunnel: w323 -> [w331 w337]
                          tunnel: w322 -> [w332 w336]
                          tunnel: [w328 w335] -> w321
                          tunnel: [w327 w334] -> w320
                          tunnel: [w326 w333] -> w319
                          frame False {
                            n192 = call "CheckFolder.vi"("Overwrite?"=w329, "Index"=w330, "File Name"=w331, "Folder Path Control"=w332) -> ("Warning"=w326:bool, "Message"=w327:string, "File Path"=w328:path)  [unwired: 5 in]
                          }
                          frame True {
                            n193 = call "CheckMonthDateFolder.vi"("Overwrite?"=w339, "Index"=w338, "File Name"=w337, "Folder Path Control"=w336) -> ("Warning"=w333:bool, "Message"=w334:string, "File Path"=w335:path)  [unwired: 5 in]
                          }
                        }
                        n194 = property on="Warning" class="Bool (strict)"("Value"=w319) -> ()  [unwired: 2 in, 2 out]
                        n195 = property on="Message" class="Str"("Value"=w320) -> ()  [unwired: 2 in, 2 out]
                      }
                    }
                  }
                  frame #5 {
                    n196 = case shown="True" w341 {
                      tunnel: w342 -> [_ w344]
                      tunnel: w340 -> [_ w343]
                      frame False {
                      }
                      frame True {
                        n197 = Not A Number/Path/Refnum?(number/path/refnum=w344) -> (NaN/Path/Refnum?=w345:bool)
                        n198 = case shown="False" w345 {
                          tunnel: w344 -> [w346 _]
                          tunnel: w343 -> [w351 _]
                          frame False {
                            # "Save Image\nand data"
                            n199 = call "SavePicture.vi"("File Path"=w346, "Image Pixels (U16)"=w351) -> ("error out"=w357:errorcluster)  [unwired: 9 in]
                            n200 = property on="Nom du fichier" class="Str"() -> ("Value"=w347:string)  [unwired: 2 in, 2 out]
                            n201 = property on="Indice" class="DigNum (strict)"() -> ("Value"=w348:u32)  [unwired: 2 in, 2 out]
                            n202 = property on="Exposure Time" class="Slide (strict)"() -> ("Value"=w349:dbl)  [unwired: 2 in, 2 out]
                            n203 = Unbundle By Name(w357) -> ("source"=w354:string, "status"=w355:bool)
                            n204 = call "FindLineAndOverwrite_Double.vi"("Exposure path"=w346, "Name"=w347, "Index"=w348, "Exposure"=w349) -> ("error out"=w350:errorcluster)  [unwired: 11 in]
                            n205 = Unbundle By Name(w350) -> ("status"=w356:bool, "source"=w358:string)
                            n206 = Or(x=w355, y=w356) -> (x .or. y?=w353:bool)
                            n207 = case shown="False" w353 {
                              tunnel: w358 -> [_ w362]
                              tunnel: w354 -> [_ w365]
                              tunnel: "\r\n" -> [_ w363]
                              frame False {
                                n208 = property on="Mode de Sauvegarde" class="Ring (strict)"() -> ("Value"=w360:u16)  [unwired: 2 in, 2 out]
                                n209 = property on="Indice" class="DigNum (strict)"() -> ("Value"=w361:u32)  [unwired: 2 in, 2 out]
                                n210 = Add(x=w361, y=w360) -> (x+y=w359:u32)
                                n211 = property on="Indice" class="DigNum (strict)"("Value"=w359) -> ()  [unwired: 2 in, 2 out]
                              }
                              frame True {
                                n212 = Concatenate Strings(w365, w363, w362) -> (w364:string)
                                n213 = property on="Message" class="Str"("Value"=w364) -> ()  [unwired: 2 in, 2 out]
                              }
                            }
                          }
                          frame True {
                          }
                        }
                      }
                    }
                  }
                }
              }
              frame Error {
              }
            }
          }
          event "Snap current Data": Value Change {
            n214 = event-data() -> ()  [unwired: 1 in, 6 out]
            n215 = stacked-sequence {
              seq-local: [w375 _] -> [_ w391]
              frame #0 {
                n216 = property on="Racine chemin de sauvegarde" class="Path"() -> ("Value"=w371:path)  [unwired: 2 in, 2 out]
                n217 = property on="Nom du fichier" class="Str"() -> ("Value"=w372:string)  [unwired: 2 in, 2 out]
                n218 = property on="Indice" class="DigNum (strict)"() -> ("Value"=w373:u32)  [unwired: 2 in, 2 out]
                n219 = property on="Overwrite?" class="Bool (strict)"() -> ("Value"=w374:bool)  [unwired: 2 in, 2 out]
                n220 = property on="Automatic\nfolder naming" class="Bool (strict)"() -> ("Value"=w368:bool)  [unwired: 2 in, 2 out]
                n221 = case shown="False" w368 {
                  tunnel: [w378 w389] -> w375
                  tunnel: w374 -> [w379 w388]
                  tunnel: w373 -> [w380 w387]
                  tunnel: w372 -> [w381 w386]
                  tunnel: w371 -> [w382 w385]
                  tunnel: [w377 w384] -> w370
                  tunnel: [w376 w383] -> w369
                  frame False {
                    n222 = call "CheckFolder.vi"("Overwrite?"=w379, "Index"=w380, "File Name"=w381, "Folder Path Control"=w382) -> ("Warning"=w376:bool, "Message"=w377:string, "File Path"=w378:path)  [unwired: 5 in]
                  }
                  frame True {
                    n223 = call "CheckMonthDateFolder.vi"("Overwrite?"=w388, "Index"=w387, "File Name"=w386, "Folder Path Control"=w385) -> ("Warning"=w383:bool, "Message"=w384:string, "File Path"=w389:path)  [unwired: 5 in]
                  }
                }
                n224 = property on="Warning" class="Bool (strict)"("Value"=w369) -> ()  [unwired: 2 in, 2 out]
                n225 = property on="Message" class="Str"("Value"=w370) -> ()  [unwired: 2 in, 2 out]
              }
              frame #1 {
                n226 = Not A Number/Path/Refnum?(number/path/refnum=w391) -> (NaN/Path/Refnum?=w390:bool)
                n227 = case shown="False" w390 {
                  tunnel: w391 -> [w395 _]
                  frame False {
                    # "Save Image\nand data"
                    n228 = property on="Captured Image" class="IntGraph (strict)"() -> ("Value"=w397:dbl[][])  [unwired: 2 in, 2 out]
                    n229 = call "SavePicture.vi"("File Path"=w395, "Image Pixels (U16)"=w397) -> ("error out"=w403:errorcluster)  [unwired: 9 in]
                    n230 = property on="Nom du fichier" class="Str"() -> ("Value"=w394:string)  [unwired: 2 in, 2 out]
                    n231 = property on="Indice" class="DigNum (strict)"() -> ("Value"=w393:u32)  [unwired: 2 in, 2 out]
                    n232 = property on="Exposure Time" class="Slide (strict)"() -> ("Value"=w392:dbl)  [unwired: 2 in, 2 out]
                    n233 = Unbundle By Name(w403) -> ("source"=w400:string, "status"=w401:bool)
                    n234 = call "FindLineAndOverwrite_Double.vi"("Exposure path"=w395, "Name"=w394, "Index"=w393, "Exposure"=w392) -> ("error out"=w396:errorcluster)  [unwired: 11 in]
                    n235 = Unbundle By Name(w396) -> ("status"=w402:bool, "source"=w404:string)
                    n236 = Or(x=w401, y=w402) -> (x .or. y?=w399:bool)
                    n237 = case shown="False" w399 {
                      tunnel: w404 -> [_ w408]
                      tunnel: w400 -> [_ w411]
                      tunnel: "\r\n" -> [_ w409]
                      frame False {
                        n238 = property on="Mode de Sauvegarde" class="Ring (strict)"() -> ("Value"=w406:u16)  [unwired: 2 in, 2 out]
                        n239 = property on="Indice" class="DigNum (strict)"() -> ("Value"=w407:u32)  [unwired: 2 in, 2 out]
                        n240 = Add(x=w407, y=w406) -> (x+y=w405:u32)
                        n241 = property on="Indice" class="DigNum (strict)"("Value"=w405) -> ()  [unwired: 2 in, 2 out]
                      }
                      frame True {
                        n242 = Concatenate Strings(w411, w409, w408) -> (w410:string)
                        n243 = property on="Message" class="Str"("Value"=w410) -> ()  [unwired: 2 in, 2 out]
                      }
                    }
                  }
                  frame True {
                  }
                }
              }
            }
          }
          event "Imager": Value Change {
            n244 = event-data() -> ()  [unwired: 1 in, 6 out]
            n245 = flat-sequence {
              tunnel: [w416] -> w412
              tunnel: w412 -> [w423]
              frame #0 {
                w414 = T1 2 items=["START_STREAM", "PAUSE_STREAM", "STOP_STREAM"] ("uStreamState IN")
                n246 = property on="Camera Handle" class="DigNum (strict)"() -> ("Value"=w413:u32)  [unwired: 2 in, 2 out]
                n247 = call <vilib>:"MEPU-Acquisition-SetStreamState.vi"("hCamera IN"=w413, "uStreamState IN"=w414) -> ("hCamera OUT"=w415:u32)  [unwired: 12 in, 1 out]
                n248 = call <vilib>:"MEPU-Initialization-Uninitialize.vi"("hCamera IN"=w415) -> ()  [unwired: 14 in, 1 out]
              }
              frame #1 {
                n249 = property on="Imager" class="Ring (strict)"() -> ("Strings []"=w421:string[], "RingText.Text"=w420:string, "StringsAndValues[]"=w418:T7)  [unwired: 2 in, 2 out]
                n250 = Search 1D Array(1D array=w421, element=w420) -> (index of element=w419:i32)  [unwired: 1 in]
                n251 = Index Array(array=w418, index=w419) -> (element=w417:cluster{"String":string, "Value":u32})
                n252 = Unbundle By Name(w417) -> ("Value"=w416:u32)
              }
              frame #2 {
                w426 = T2 1 items=["FEATURE_FLAG_PRESENCE                 0x00000001", "FEATURE_FLAG_MANUAL                     0x00000002", "FEATURE_FLAG_AUTO                         0x00000004", "FEATURE_FLAG_ONEPUSH                   0x00000008", "FEATURE_FLAG_OFF                            0x00000010", "FEATURE_FLAG_DESC_SUPPORTED    0x00000020", "FEATURE_FLAG_READ_ONLY               0x00000040"] ("uFlags IN")
                w425 = T3 8 items=["FEATURE_BRIGHTNESS", "FEATURE_EXPOSURE", "FEATURE_SHARPNESS", "FEATURE_WHITE_BAL", "FEATURE_HUE", "FEATURE_SATURATION", "FEATURE_GAMMA", "FEATURE_SHUTTER", "FEATURE_GAIN", "FEATURE_IRIS", "FEATURE_FOCUS", "FEATURE_TEMPERATURE", "FEATURE_TRIGGER", "FEATURE_ZOOM", "FEATURE_PAN", "FEATURE_TILT", "FEATURE_OPT_FILTER", "FEATURE_GPIO", "FEATURE_FRAME_RATE", "FEATURE_ROI", "FEATURE_FLIP", "FEATURE_PIXEL_ADDRESSING", "FEATURE_PIXEL_FORMAT", "FEATURE_EXTENDED_SHUTTER", "FEATURE_AUTO_ROI", "FEATURE_LOOKUP_TABLE", "FEATURE_MEMORY_CHANNEL", "FEATURE_WHITE_SHADING", "FEATURE_ROTATE", "FEATURE_IMAGER_CLK_DIVISOR", "FEATURE_TRIG_WITH_CNTRLD_LIGHT", "FEATURE_MAX_PIXEL_SIZE"] ("uFeatureId IN")
                w432 = T2 1 items=["FEATURE_FLAG_PRESENCE                 0x00000001", "FEATURE_FLAG_MANUAL                     0x00000002", "FEATURE_FLAG_AUTO                         0x00000004", "FEATURE_FLAG_ONEPUSH                   0x00000008", "FEATURE_FLAG_OFF                            0x00000010", "FEATURE_FLAG_DESC_SUPPORTED    0x00000020", "FEATURE_FLAG_READ_ONLY               0x00000040"] ("uFlags IN")
                w433 = T3 22 items=["FEATURE_BRIGHTNESS", "FEATURE_EXPOSURE", "FEATURE_SHARPNESS", "FEATURE_WHITE_BAL", "FEATURE_HUE", "FEATURE_SATURATION", "FEATURE_GAMMA", "FEATURE_SHUTTER", "FEATURE_GAIN", "FEATURE_IRIS", "FEATURE_FOCUS", "FEATURE_TEMPERATURE", "FEATURE_TRIGGER", "FEATURE_ZOOM", "FEATURE_PAN", "FEATURE_TILT", "FEATURE_OPT_FILTER", "FEATURE_GPIO", "FEATURE_FRAME_RATE", "FEATURE_ROI", "FEATURE_FLIP", "FEATURE_PIXEL_ADDRESSING", "FEATURE_PIXEL_FORMAT", "FEATURE_EXTENDED_SHUTTER", "FEATURE_AUTO_ROI", "FEATURE_LOOKUP_TABLE", "FEATURE_MEMORY_CHANNEL", "FEATURE_WHITE_SHADING", "FEATURE_ROTATE", "FEATURE_IMAGER_CLK_DIVISOR", "FEATURE_TRIG_WITH_CNTRLD_LIGHT", "FEATURE_MAX_PIXEL_SIZE"] ("uFeatureId IN")
                n253 = call <vilib>:"MEPU-Initialization-InitializeSystem.vi"() -> ("Error OUT"=w439:errorcluster)  [unwired: 15 in]
                n254 = control-ref of="Exposure Time"() -> (w438:refnum<vi>)
                n255 = call <vilib>:"MEPU-Initialization-Initialize.vi"("uSerialNumber IN"=w423, "Error IN"=w439) -> ("phCamera OUT"=w437:u32, "Error OUT"=w436:errorcluster)  [unwired: 11 in, 1 out]
                n256 = call "Setup Exposure.vi"("Error IN"=w436, "Shutter"=w438, "hCamera IN"=w437) -> ("Error OUT"=w435:errorcluster, "phCamera OUT"=w434:u32)  [unwired: 7 in]
                n257 = Build Array(1.0) -> (w430:dbl[])
                n258 = call <vilib>:"MEPU-CameraFeatures-SetFeature.vi"("hCamera IN"=w434, "uFeatureId IN"=w433, "uFlags IN"=w432, "pParms IN"=w430, "Error IN"=w435) -> ("hCamera OUT"=w424:u32, "Error OUT"=w429:errorcluster)  [unwired: 8 in, 1 out]
                n259 = Build Array(0.0) -> (w427:dbl[])
                n260 = call <vilib>:"MEPU-CameraFeatures-SetFeature.vi"("hCamera IN"=w424, "uFeatureId IN"=w425, "uFlags IN"=w426, "pParms IN"=w427, "Error IN"=w429) -> ("hCamera OUT"=w422:u32)  [unwired: 8 in, 2 out]
                n261 = property on="Camera Handle" class="DigNum (strict)"("Value"=w422) -> ()  [unwired: 2 in, 2 out]
              }
            }
          }
        }
      }
      n262 = property on="Error OUT" class="Clust (strict)"("Value"=w67) -> ()  [unwired: 2 in, 2 out]
    }
    frame #4 {
      w442 = T1 2 items=["START_STREAM", "PAUSE_STREAM", "STOP_STREAM"] ("uStreamState IN")
      # "Ignore errors here to ensure as\ncomplete a clean up as possible."
      n263 = property on="Camera Handle" class="DigNum (strict)"() -> ("Value"=w440:u32)  [unwired: 2 in, 2 out]
      n264 = call <vilib>:"MEPU-Acquisition-SetStreamState.vi"("hCamera IN"=w440, "uStreamState IN"=w442) -> ("hCamera OUT"=w444:u32)  [unwired: 12 in, 1 out]
      n265 = call <vilib>:"MEPU-Initialization-Uninitialize.vi"("hCamera IN"=w444) -> ("Error OUT"=w443:errorcluster)  [unwired: 14 in]
      n266 = stacked-sequence {
        tunnel: w443 -> [_]
        frame #0 {
          n267 = call <vilib>:"MEPU-Initialization-UninitializeSystem.vi"() -> ()  [unwired: 15 in, 1 out]
        }
      }
    }
  }
  n268 = Or(x=w3, y=w2) -> (x .or. y?=w1:bool)
  n269 = property on="stop" class="Bool (strict)"("Value"=w1) -> ()  [unwired: 2 in, 2 out]
